vi "mod_Bits to Message String.vi"(0 "input bit stream":i8[](array[numeric])) -> (4 "message string":string)   [LabVIEW 2020, in "niDMT.lvlib"]
uses:
  <vilib>/addons/Modulation/niDMT.lvlib
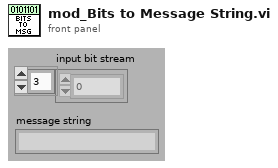
[diagram p1: front panel]
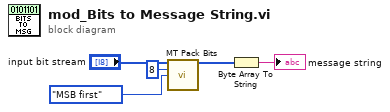
[diagram p0: block diagram]
diagram:
  n1 = call <vilib>:"MT Pack Bits.vi"("input bit stream"="input bit stream", "bits per integer"=8, "packed bit order"=enum16{"MSB first", "LSB first"}."MSB first") -> ("output integers"=w2:i32[])  [unwired: 3 in, 9 out]
  n2 = Byte Array To String(unsigned byte array=w2) -> (string=→"message string":string)
